vi "PH_Beckhoff_PP_PU.set Safe State.vi"(0 "i ref in":refnum<vi>, 5 "error in":errorcluster) -> (14 "i ref out":refnum<vi>, 19 "error out":errorcluster)   [LabVIEW 2014, in "PH_Beckhoff_PP_PU.lvlib"]
doc: "This VI calls several simple event calls to set the hardware to a safe (default) state. It is supposed to be used in con- and destructor."
uses:
  PH_Beckhoff_PP_PU.lvlib
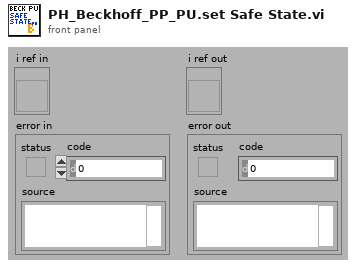
[diagram p1: front panel]
types:
  T1 = typedef "PH_Beckhoff_PP_PU.lvlib/PH_Beckhoff_PP_PU.PU Rack Type.ctl" = enum16{"no Info", "PA 19mm", "PA 45mm", "MA PU 1 and 2", "MA PU 3 and 4", "MA PU 5 and 6", "MA FR and PILC"}
  T2 = typedef "PH_PP_Common.lvlib/PH_PP_Common.PUs.ctl" = enum16{"no Info", "PA-19mm-1", "PA-19mm-2", "PA-45mm-PILC", "PA-45mm-MAIN", "MA-PU-1", "MA-PU-2", "MA-PU-3", "MA-PU-4", "MA-PU-5", "MA-PU-6", "MA-FR", "MA-PILC", "PA-45mm-DP"}
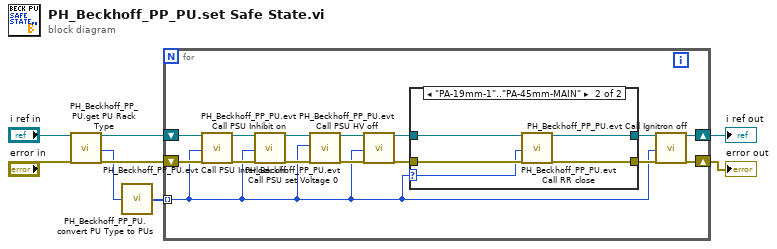
[diagram p0: block diagram]
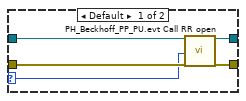
[diagram p2: hidden frame]
diagram:
  n1 = call "PH_Beckhoff_PP_PU.get PU Rack Type.vi"("VI in"="i ref in", "error in (no error)"="error in") -> ("VI out"=w5:refnum<vi>, "PU Rack Type"=w1:T1, "error out"=w6:errorcluster)  [unwired: 15 in]
  n2 = call "PH_Beckhoff_PP_PU.convert PU Type to PUs.vi"("PU Type"=w1) -> ("PUs"=w4:T2[])
  n3 = for {
    shift-right: [w13] -> w7
    shift-left: w6 -> [w19]
    shift-right: [w11] -> w3
    shift-left: w5 -> [w15]
    tunnel: w4 -> [w9] mode=indexing
    n4 = call "PH_Beckhoff_PP_PU.evt Call PSU Inhibit on.vi"("i ref in"=w15, "PU"=w9, "error in"=w19) -> ("i ref out"=w18:refnum<vi>, "error out"=w22:errorcluster)  [unwired: 15 in]
    n5 = call "PH_Beckhoff_PP_PU.evt Call PSU Interlock off.vi"("i ref in"=w18, "PU"=w9, "error in"=w22) -> ("i ref out"=w17:refnum<vi>, "error out"=w23:errorcluster)  [unwired: 15 in]
    n6 = call "PH_Beckhoff_PP_PU.evt Call PSU set Voltage 0.vi"("i ref in"=w17, "PU"=w9, "error in"=w23) -> ("i ref out"=w16:refnum<vi>, "error out"=w21:errorcluster)  [unwired: 15 in]
    n7 = call "PH_Beckhoff_PP_PU.evt Call PSU HV off.vi"("i ref in"=w16, "PU"=w9, "error in"=w21) -> ("i ref out"=w14:refnum<vi>, "error out"=w20:errorcluster)  [unwired: 15 in]
    n8 = case shown="\"PA-19mm-1\"..\"PA-45mm-MAIN\"" w9 {
      selector: w9 -> [w26 w31]
      tunnel: w20 -> [w28 w33]
      tunnel: [w24 w29] -> w12
      tunnel: w14 -> [w27 w32]
      tunnel: [w25 w30] -> w10
      frame Default {
        n9 = call "PH_Beckhoff_PP_PU.evt Call RR open.vi"("i ref in"=w27, "PU"=w26, "error in"=w28) -> ("i ref out"=w25:refnum<vi>, "error out"=w24:errorcluster)  [unwired: 15 in]
      }
      frame "PA-19mm-1".."PA-45mm-MAIN" {
        n10 = call "PH_Beckhoff_PP_PU.evt Call RR close.vi"("i ref in"=w32, "PU"=w31, "error in"=w33) -> ("i ref out"=w30:refnum<vi>, "error out"=w29:errorcluster)  [unwired: 15 in]
      }
    }
    n11 = call "PH_Beckhoff_PP_PU.evt Call Ignitron off.vi"("i ref in"=w10, "PU"=w9, "error in"=w12) -> ("i ref out"=w11:refnum<vi>, "error out"=w13:errorcluster)  [unwired: 15 in]
  }
  "i ref out" <- w3
  "error out" <- w7
